vi "RunMe (Test Launcher).vi"() -> ()   [LabVIEW 2020, in "Caraya.lvlib" / "Test Runner.Template.lvclass"]
uses:
  Test Runner.Template.lvclass
  C:/projects/caraya/src/classes/Test Runner/Test Runner.lvclass
  Test Runner/Test Runner.lvclass
panel:
  out "error out":errorcluster
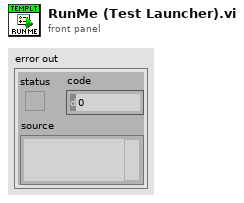
[diagram p1: front panel]
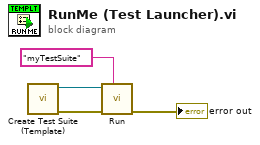
[diagram p0: block diagram]
diagram:
  n1 = call "Create Test Suite (Template).vi"() -> ("error out"=w3:errorcluster, "Test Runner.Template out"=w4:refnum<class "Test Runner.Template.lvclass">)  [unwired: 10 in]
  n2 = call "Run.vi"("Name"="myTestSuite", "error in (no error)"=w3, "Test Runner in"=w4) -> ("error out"=→"error out":errorcluster)  [unwired: 6 in, 2 out]
